vi "weideman64.vi"(9 "imag_in":dbl, 10 "real_in":dbl) -> (2 "imag_out":dbl, 3 "real_out":dbl)   [LabVIEW 2022 SP3]
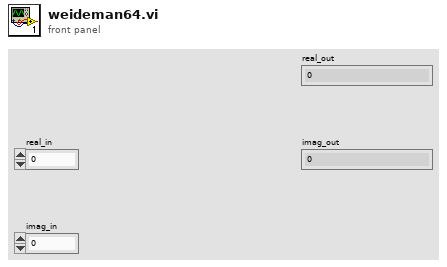
[diagram p1: front panel]
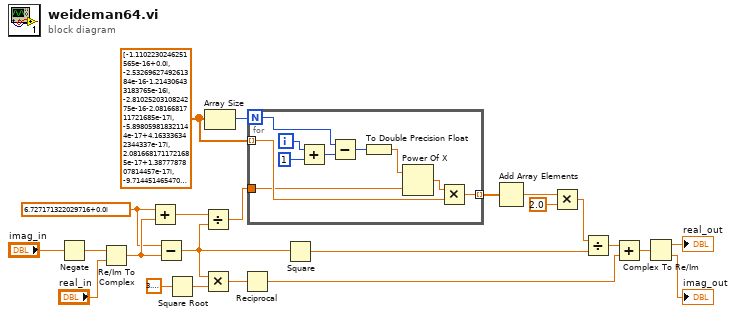
[diagram p0: block diagram]
diagram:
  w1 = cdb 6.727171322029716+0.0i ("double precision complex")
  w2 = cdb[] [-1.1102230246251565e-16+0.0i, -2.5326962749261384e-16-1.214306433183765e-16i, -2.8102520310824275e-16-2.0816681711721685e-17i, -5.898059818321144e-17+4.163336342344337e-17i, 2.0816681711721685e-17+1.3877787807814457e-17i, -9.71445146547012e-17+1.5265566588595902e-16i, -1.5265566588595902e-16+1.457167719820518e-16i, -1.1102230246251565e-16+1.231653667943533e-16i, -3.8163916471489756e-17+2.0816681711721685e-17i, -1.8453120975703285e-16+2.6020852139652106e-17i, -3.209238430557093e-17+4.423544863740858e-17i, -4.5102810375396984e-17+2.6454533008646308e-17i, -1.3010426069826053e-18+4.7704895589362195e-17i, -8.782037597132586e-17+9.107298248878237e-18i, 4.0007060164715114e-17+2.0491421059976034e-17i, 2.3960868011929648e-17+4.9060148304969076e-18i, 7.632783294297951e-17-4.3368086899420173e-19i, 2.168404344971009e-17+4.8468213806792854e-17i, 2.42861286636753e-17-3.9114552886268407e-17i, -1.0489656018797255e-17+1.2439806394283322e-16i, 1.8709263738952986e-16+4.527122932099158e-17i, 3.3148634390797044e-16+3.941426939411514e-18i, -8.463518996774834e-16+7.477055560139036e-17i, -4.382651383596841e-15-5.95638692098458e-17i, -2.8079105143788614e-16-2.4532694666933983e-18i, 3.2856216329850435e-14+5.441974978023115e-19i, 5.898216965928481e-14+2.369086567458805e-17i, -1.5485679457460615e-13-6.294317714168243e-17i, -7.921876070347195e-13-1.4719616800160393e-17i, -3.9394220371261186e-13+1.0633241606016208e-16i, 5.8326573542676235e-12+1.8712109230856848e-17i, 1.7501521550594263e-11+8.571999631358013e-17i, -6.470633436423956e-12+0.0i, -1.7560600195747912e-10+2.5302306148935514e-17i, -4.533914545493771e-10+9.231019323165881e-17i, 2.44348066206543e-10+5.0676829808215436e-17i, 5.186955662307426e-09-6.378500613402836e-17i, 1.592681408652797e-08-1.556144579250633e-17i, 7.4357107773048325e-09-2.369086567458805e-17i, -1.3610261241433205e-07+1.5714642266361136e-17i, -6.650424120091667e-07-1.7172886266853793e-17i, -1.5547722782696825e-06-4.669632933997187e-17i, -7.564244112633297e-08-3.697958577626202e-18i, 1.790180158612915e-05-1.0123037661480153e-16i, 0.00010227006798910055+5.811478526595972e-17i, 0.0003962745103980495+6.176154548448746e-17i, 0.0012549788049981822+1.833397992971893e-17i, 0.0034602079481074804-6.761439709735201e-19i, 0.008565381413175907+2.168404344971009e-19i, 0.019380399024538218-3.233632979438017e-17i, 0.04055284652958023+8.088148206741863e-17i, 0.07911655067602588-1.951563910473908e-18i, 0.1447785997358641+6.982261990806649e-17i, 0.24963969994535562-6.028164079019405e-17i, 0.4070443030398736+9.8879238130678e-17i, 0.6293868343374367-2.3852447794681098e-18i, 0.9249760252638086+3.122502256758253e-17i, 1.2944377517175158+8.500145032286355e-17i, 1.7275060857871172+7.632783294297951e-17i, 2.20125657128641+2.7755575615628914e-17i, 2.680732639559084+2.0816681711721685e-17i, 3.1224481894020366+7.28583859910259e-17i, 3.4804961039850415+1.0408340855860843e-17i, 3.7141697931977022-1.3183898417423734e-16i] ("reversed array")
  n1 = Negate(x="imag_in") -> (-x=w22:dbl)
  n2 = Re/Im To Complex(1:"real_in", 2:w22) -> (0:w20:cdb)
  n3 = Add(x=w1, y=w20) -> (x+y=w4:cdb)
  n4 = Subtract(x=w1, y=w20) -> (x-y=w13:cdb)
  n5 = Square Root(x=3.141592653589793) -> (sqrt(x)=w14:dbl)
  n6 = Divide(x=w4, y=w13) -> (x/y=w3:cdb)
  n7 = Multiply(x=w13, y=w14) -> (x*y=w7:cdb)
  n8 = Array Size(array=w2) -> (size(s)=w19:i32)
  n9 = Reciprocal(x=w7) -> (1/x=w6:cdb)
  n10 = for {
    N: w19 -> [w33]
    tunnel: w2 -> [w32] mode=indexing
    tunnel: w3 -> [w25]
    tunnel: [w31] -> w18 mode=indexing
    i -> [w29]
    n11 = Add(x=w29, y=1 ("x")) -> (x+y=w28:i32)
    n12 = Subtract(x=w33, y=w28) -> (x-y=w26:i32)
    n13 = To Double Precision Float(number=w26) -> (double precision float=w24:dbl)
    n14 = Power Of X(1:w25, 2:w24) -> (0:w27:cdb)
    n15 = Multiply(x=w27, y=w32) -> (x*y=w31:cdb)
  }
  n16 = Square(x=w13) -> (x^2=w9:cdb)
  n17 = Add Array Elements(numeric array=w18) -> (sum=w12:cdb)
  n18 = Multiply(x=w12, y=2.0 ("x")) -> (x*y=w10:cdb)
  n19 = Divide(x=w10, y=w9) -> (x/y=w8:cdb)
  n20 = Add(x=w8, y=w6) -> (x+y=w5:cdb)
  n21 = Complex To Re/Im(x + iy=w5) -> (x=→"real_out":dbl, y=→"imag_out":dbl)
